vi "VIToRun.vi"() -> ()   [LabVIEW 2013]
panel:
  in  "Base":dbl format="%.2f"
  in  "Numeric Input Value":dbl format="%.2f"
  out "Numeric Output Value":dbl format="%.2f"
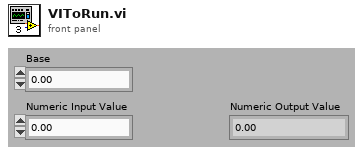
[diagram p1: front panel]
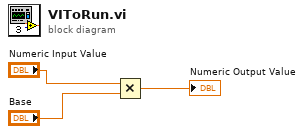
[diagram p0: block diagram]
diagram:
  n1 = Multiply(x="Numeric Input Value", y="Base") -> (x*y=→"Numeric Output Value":dbl)
